vi "gfitsio-write-key-string.vi"(6 "comment":string, 7 "keyname":string, 8 "error in (no error)":errorcluster, 9 "value":string, 11 "gfits refnum":T1) -> (0 "error out":errorcluster, 3 "dup gfits refnum":T1)   [LabVIEW 2023, in "gfitsio.lvlib"]
doc: "Write a keyword of the appropriate data type into the current HDU. If the keyword already exists it will be overwritten. Otherwise a new keyword will be appended to the header."
uses:
  gfitsio.lvlib
  cfitsio-datatypes.ctl
  gfitsio.dll
  gfitsio-refnum.ctl
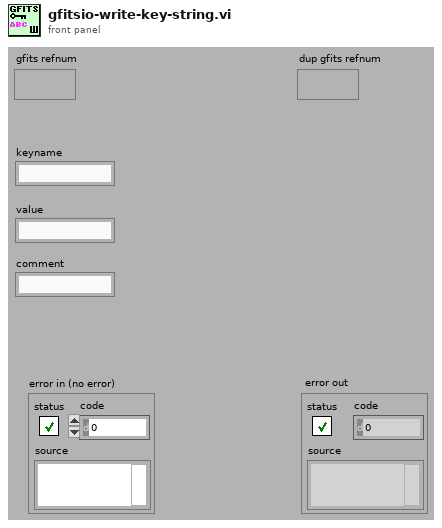
[diagram p1: front panel]
types:
  T1 = typedef "gfitsio.lvlib/gfitsio-refnum.ctl" = refnum<k1>
  T2 = typedef "gfitsio.lvlib/cfitsio-datatypes.ctl" = i32
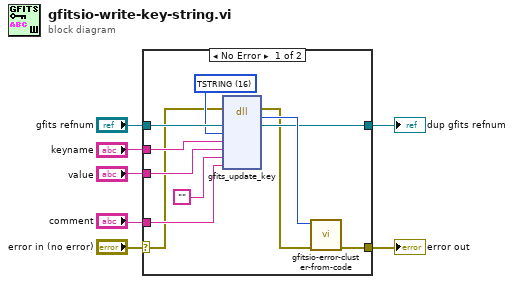
[diagram p0: block diagram]
diagram:
  n1 = case shown="No Error" "error in (no error)" {
    selector: "error in (no error)" -> [w8 w20]
    tunnel: [w17 w20] -> w1
    tunnel: "gfits refnum" -> [w15 w19]
    tunnel: [w16 w19] -> w6
    tunnel: "keyname" -> [w13 _]
    tunnel: "value" -> [w12 _]
    tunnel: "comment" -> [w11 _]
    frame No Error {
      w14 = T2 16 items=["TBIT"=1, "TBYTE  (U8)"=11, "TSBYTE  (I8)"=12, "TLOGICAL"=14, "TSTRING"=16, "TUSHORT  (U16)"=20, "TSHORT  (I16)"=21, "TUINT"=31, "TULONG  (U32)"=40, "TLONG  (I32)"=41, "TFLOAT  (SGL)"=42, "TLONGLONG  (I64)"=81, "TDOUBLE  (DBL)"=82, "TCOMPLEX  (CSG)"=83, "TDOUBLECOMPLEX  (CDB)"=163] ("cfitsio datatype")
      n2 = dll-call lib="gfitsio.dll" fn="gfits_update_key"(error in=w8, "refnum"=w15, "datatype"=w14, "keyname"=w13, "value"=w12, "unit"="", "comment"=w11) -> (error out=w9:errorcluster, w18:i32, "refnum"=w16:T1)  [unwired: 6 in, 2 out]
      n3 = call "gfitsio-error-cluster-from-code.vi"("error in (no error)"=w9, "error code"=w18) -> ("error out"=w17:errorcluster)  [unwired: 9 out]
    }
    frame Error {
    }
  }
  "error out" <- w1
  "dup gfits refnum" <- w6
